vi "get_config_cluster.vi"(8 "error in (no error)":errorcluster, 11 "GenericPlugin in":refnum<class "ComponentTemplate.lvclass">) -> (0 "error out":errorcluster, 2 "config cluster (variant)":variant, 3 "GenericPlugin out":refnum<class "ComponentTemplate.lvclass">)   [LabVIEW 2010]
uses:
  ComponentTemplate.lvclass
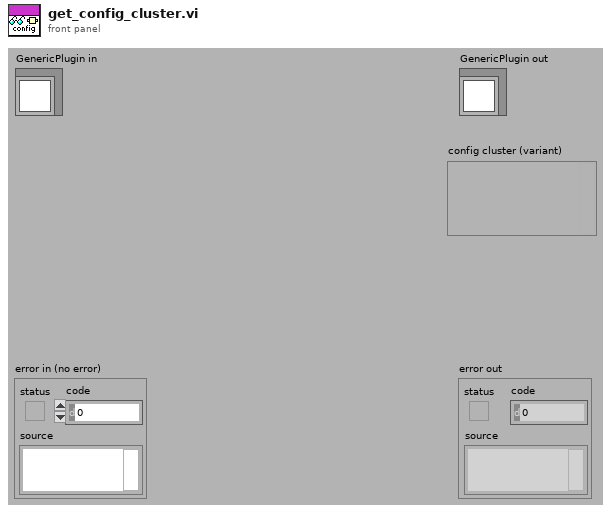
[diagram p1: front panel]
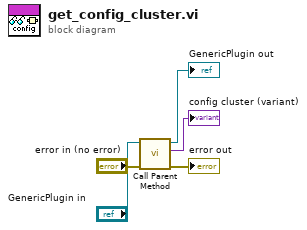
[diagram p0: block diagram]
diagram:
  n1 = call-parent "Call Parent Method"("error in (no error)"="error in (no error)", "GenericComponent in"="GenericPlugin in") -> ("error out"=→"error out":errorcluster, "config cluster (variant)"=→"config cluster (variant)":variant, "GenericComponent out"=→"GenericPlugin out":refnum<class "ComponentTemplate.lvclass">)  [unwired: 7 in]
